vi "Read Problem.vi"(8 "error in (no error)":errorcluster, 11 "file path (use dialog)":path=path "") -> (0 "error out":errorcluster, 3 "svm_problem":T1)   [LabVIEW 2014]
doc: "Reads a file containing libsvm-formatted training data. For example from the data sets page on the official libsvm page."
uses:
  LibSVM Sparse/Wrapper API/Controls/svm_problem.ctl
  LibSVM Sparse/Wrapper API/Controls/svm_node.ctl
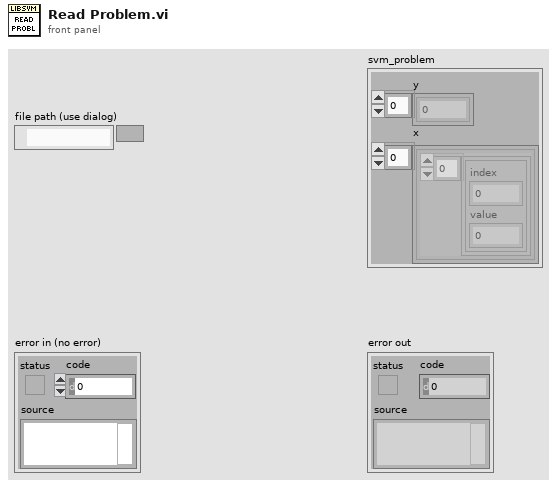
[diagram p1: front panel]
types:
  T1 = typedef "svm_problem.ctl" = cluster{"y":dbl[], "x":cluster{T2[]}[]}
  T2 = typedef "svm_node.ctl" = cluster{"index":i32, "value":dbl}
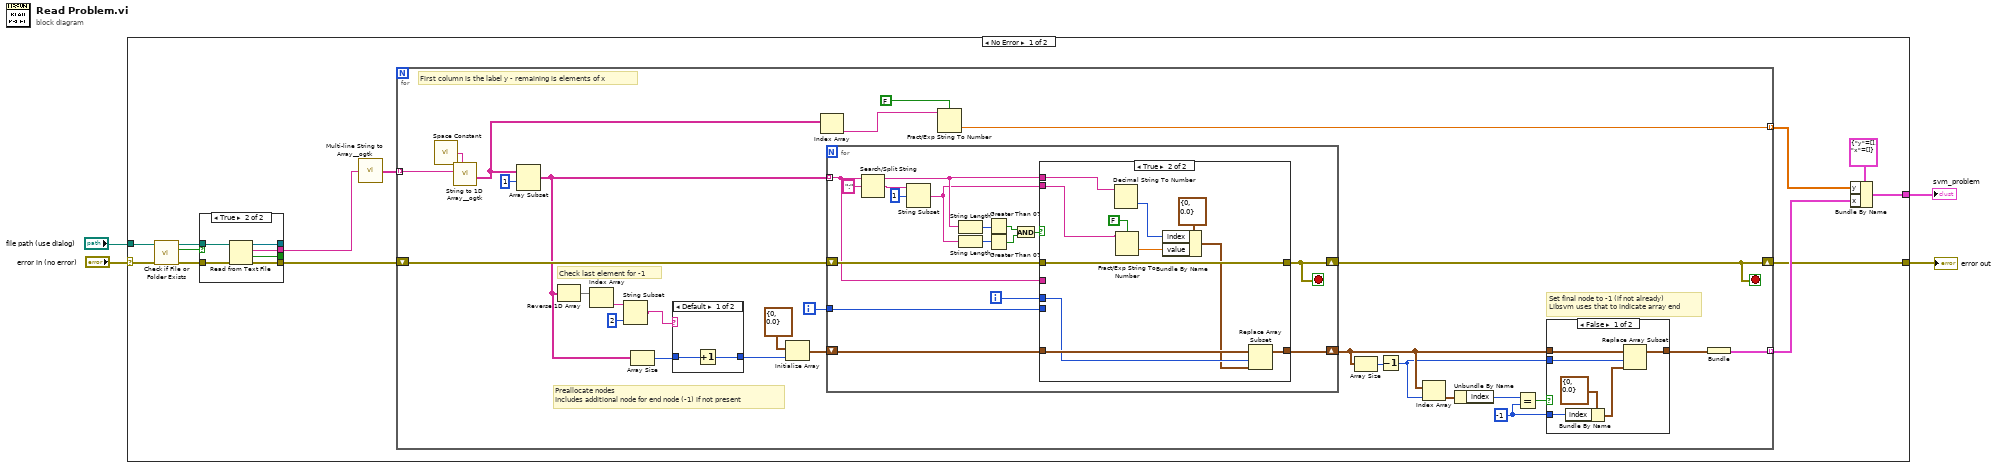
[diagram p0: block diagram]
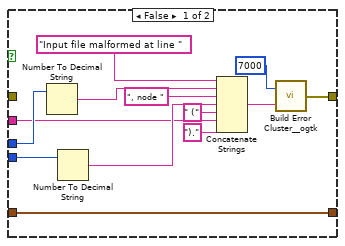
[diagram p4: hidden frame]
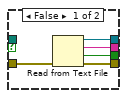
[diagram p5: hidden frame]
diagram:
  n1 = case shown="No Error" "error in (no error)" {
    selector: "error in (no error)" -> [w17 w108]
    tunnel: [w5 w108] -> w4
    tunnel: "file path (use dialog)" -> [w15 _]
    tunnel: [w6 _] -> w1
    frame No Error {
      n2 = call <vilib>:"Check if File or Folder Exists.vi"("error in (no error)"=w17, "path"=w15) -> ("error out"=w16:errorcluster, "file or folder exists?"=w14:bool, "dup path"=w13:path)  [unwired: 7 in]
      n3 = case shown="True" w14 {
        tunnel: w16 -> [w101 w107]
        tunnel: w13 -> [_ w105]
        tunnel: [w100 w106] -> w11
        tunnel: [w99 w104] -> _
        tunnel: [w98 w103] -> _
        tunnel: [w97 w102] -> w12
        frame False {
          n4 = Read from Text File(error in=w101) -> (refnum out=w99:refnum<file>, text=w97:string, cancelled=w98:bool, error out=w100:errorcluster)  [unwired: 3 in]
        }
        frame True {
          n5 = Read from Text File(file (use dialog)=w105, error in=w107) -> (refnum out=w104:refnum<file>, text=w102:string, cancelled=w103:bool, error out=w106:errorcluster)  [unwired: 2 in]
        }
      }
      n6 = call <userlib>:"Multi-line String to Array__ogtk.vi"("string"=w12) -> ("lines"=w10:string[])
      n7 = for {
        tunnel: w10 -> [w45] mode=indexing
        tunnel: [w41] -> w7 mode=indexing
        tunnel: [w38] -> w8 mode=indexing
        shift-right: [w37] -> w5
        shift-left: w11 -> [w40]
        i -> [w39]
        stop <- w37 stop-if-true
        w25 = -1 ("y")
        # "Check last element for -1"
        # "Set final node to -1 (if not already)\nLibsvm uses that to indicate array end"
        # "Preallocate nodes\nIncludes additional node for end node (-1) if not present"
        # "First column is the label y - remaining is elements of x"
        n8 = call <vilib>:"Space Constant.vi"() -> ("String"=w44:string)
        n9 = call <userlib>:"String to 1D Array__ogtk.vi"("delimiter (Tab)"=w44, "string"=w45) -> ("Array of Strings"=w35:string[])  [unwired: 9 in]
        n10 = Array Subset(array=w35, index=1) -> (w18:string[])  [unwired: 1 in]
        n11 = Reverse 1D Array(array=w18) -> (reversed array=w24:string[])
        n12 = Index Array(array=w24) -> (element=w23:string)  [unwired: 1 in]
        n13 = String Subset(string=w23, length (rest)=2 ("length (rest)")) -> (substring=w21:string)  [unwired: 1 in]
        n14 = Array Size(array=w18) -> (size(s)=w20:i32)
        n15 = case shown="Default" w21 {
          tunnel: w20 -> [w46 w48]
          tunnel: [w47 w48] -> w19
          frame Default {
            n16 = Increment(x=w46) -> (x+1=w47:i32)
          }
          frame "-1" {
          }
        }
        n17 = Initialize Array(T2 {"index"=0, "value"=0.0} ("svm_node"), w19) -> (w33:T2[])
        n18 = Index Array(array=w35) -> (element=w43:string)  [unwired: 1 in]
        n19 = for {
          tunnel: w18 -> [w65] mode=indexing
          tunnel: w39 -> [w57]
          shift-right: [w62] -> w37
          shift-left: w40 -> [w67]
          shift-right: [w63] -> w30
          shift-left: w33 -> [w56]
          i -> [w66]
          stop <- w62 stop-if-true
          n20 = Search/Split String(string=w65, search string/char (-)=":") -> (substring before match=w64:string, match + rest of string=w60:string)  [unwired: 1 in, 1 out]
          n21 = String Subset(string=w60, offset (0)=1) -> (substring=w58:string)  [unwired: 1 in]
          n22 = String Length(string=w64) -> (length=w61:i32)
          n23 = String Length(string=w58) -> (length=w71:i32)
          n24 = Greater Than 0?(x=w61) -> (x > 0?=w70:bool)
          n25 = Greater Than 0?(x=w71) -> (x > 0?=w69:bool)
          n26 = And(x=w70, y=w69) -> (x .and. y?=w68:bool)
          n27 = case shown="True" w68 {
            tunnel: w67 -> [_ w96]
            tunnel: [w84 w96] -> w62
            tunnel: w66 -> [w83 w90]
            tunnel: w57 -> [w82 _]
            tunnel: w65 -> [w75 _]
            tunnel: w64 -> [_ w94]
            tunnel: w58 -> [_ w93]
            tunnel: [w73 w92] -> w63
            tunnel: w56 -> [w73 w91]
            frame False {
              n28 = Number To Decimal String(number=w83) -> (decimal integer string=w80:string)  [unwired: 1 in]
              n29 = Number To Decimal String(number=w82) -> (decimal integer string=w78:string)  [unwired: 1 in]
              n30 = Concatenate Strings("Input file malformed at line " ("String to Prepend to source (\"\")"), w80, ", node " ("string"), w78, " (" ("string"), w75, ")." ("string")) -> (w74:string)
              n31 = call <userlib>:"Build Error Cluster__ogtk.vi"("String to Prepend to source (\"\")"=w74, "code"=7000) -> ("error out"=w84:errorcluster)
            }
            frame True {
              n32 = Decimal String To Number(string=w94) -> (number=w86:i32)  [unwired: 2 in, 1 out]
              n33 = Fract/Exp String To Number(use system decimal point (T)=FALSE, string=w93) -> (number=w87:dbl)  [unwired: 2 in, 1 out]
              n34 = Bundle By Name(cluster=T2 {"index"=0, "value"=0.0} ("svm_node"), "index"=w86, "value"=w87) -> (w88:T2)
              n35 = Replace Array Subset(array=w91, new element=w88, index=w90) -> (w92:T2[])
            }
          }
        }
        n36 = Fract/Exp String To Number(use system decimal point (T)=FALSE, string=w43) -> (number=w41:dbl)  [unwired: 2 in, 1 out]
        n37 = Array Size(array=w30) -> (size(s)=w31:i32)
        n38 = Decrement(x=w31) -> (x-1=w26:i32)
        n39 = Index Array(array=w30, index=w26) -> (element=w29:T2)
        n40 = Unbundle By Name(w29) -> ("index"=w28:i32)
        n41 = Equal?(x=w28, y=w25) -> (x = y?=w27:bool)
        n42 = case shown="False" w27 {
          tunnel: [w54 w55] -> w32
          tunnel: w30 -> [w53 w55]
          tunnel: w26 -> [w52 _]
          tunnel: w25 -> [w50 _]
          frame False {
            n43 = Bundle By Name(cluster=T2 {"index"=0, "value"=0.0} ("svm_node"), "index"=w50) -> (w49:T2)
            n44 = Replace Array Subset(array=w53, new element=w49, index=w52) -> (w54:T2[])
          }
          frame True {
          }
        }
        n45 = Bundle(w32) -> (w38:cluster{T2[]})  [unwired: 1 in]
      }
      n46 = Bundle By Name(cluster=T1 {"y"=[], "x"=[]} ("svm_problem"), "y"=w7, "x"=w8) -> (w6:T1)
    }
    frame Error {
    }
  }
  "error out" <- w4
  "svm_problem" <- w1
